vi "dfd_FXP PtByPt Cascaded SOS Form II.vi"(0 "x":T1={"value"=0, "wl"=0, "iwl"=0, "Signed"=TRUE} {"value" format="%.0x"}, 1 "coef b":i64[](array[numeric]), 2 "coef a":i64[](array[numeric]), 3 "#sec":i32, 5 "filtering statistics in":T4(array[cluster]) {"statistics information"."min value" format="%.2f"; "statistics information"."max value" format="%.2f"; "Quantizer Source" items=["Coefficients a/k"=0, "Coefficients b/v"=7, "Input"=1, "Output"=2, "Multiplicand"=3, "Product"=4, "Sum"=5, "Delay"=6]}, 6 "quantizers":T5[](array[typedef]) {"source" items=["Coef a/k"=0, "Coef b/v"=7, "Input"=1, "Output"=2, "Multiplicand"=3, "Product"=4, "Sum"=5, "Delay"=6, "Gain"=8]}, 7 "state in":i64[](array[numeric])) -> (13 "state out":i64[](array[numeric]), 14 "filtered x":T1={"value"=0, "wl"=0, "iwl"=0, "Signed"=TRUE} {"value" format="%.0x"}, 19 "filtering statistics out":T4(array[cluster]) {"statistics information"."min value" format="%.2f"; "statistics information"."max value" format="%.2f"; "Quantizer Source" items=["Coefficients a/k"=0, "Coefficients b/v"=7, "Input"=1, "Output"=2, "Multiplicand"=3, "Product"=4, "Sum"=5, "Delay"=6]})   [LabVIEW 2017, in "NI_DigFilter_FXP.lvlib"]
uses:
  <vilib>/addons/Digital Filter Design/NI_DigFilter_FXP.lvlib
  <vilib>/addons/Digital Filter Design/_Objects.llb/dfd_DFXP Data Type (scaler).ctl
  <vilib>/addons/Digital Filter Design/_Objects.llb/dfd_DFXP Operation Parameter.ctl
  <vilib>/addons/Digital Filter Design/_Objects.llb/dfd_Internal Quantization Srcs.ctl
  <vilib>/addons/Digital Filter Design/_Objects.llb/DFD Quantization Sources.ctl
  <vilib>/addons/Digital Filter Design/_Objects.llb/DFD FXP Statistics Data.ctl
  <vilib>/addons/Digital Filter Design/NI_DigFilterLicensed.lvlib
panel:
  in  "coef_a":T1={"value"=0, "wl"=0, "iwl"=0, "Signed"=TRUE} {"value" format="%.0x"}
  in  "coef_b":T1={"value"=0, "wl"=0, "iwl"=0, "Signed"=TRUE} {"value" format="%.0x"}
  in  "state":T1={"value"=0, "wl"=0, "iwl"=0, "Signed"=TRUE} {"value" format="%.0x"}
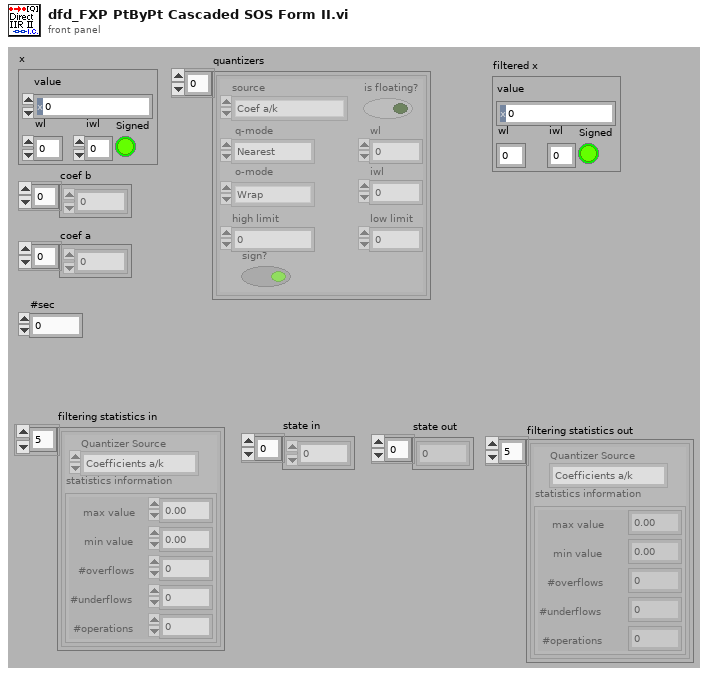
[diagram p1: front panel]
types:
  T1 = typedef "dfd_DFXP Data Type (scaler).ctl" = cluster{"value":i64, "wl":i16, "iwl":i16, "Signed":bool}
  T2 = typedef "NI_DigFilterLicensed.lvlib/DFD Quantization Sources.ctl" = u16
  T3 = typedef "NI_DigFilterLicensed.lvlib/DFD FXP Statistics Data.ctl" = cluster{"max value":ext, "min value":ext, "#overflows":i32, "#underflows":i32, "#operations":i32}
  T4 = cluster{"Quantizer Source":T2, "statistics information":T3}[]
  T5 = typedef "dfd_DFXP Operation Parameter.ctl" = cluster{"source":T6, "is floating?":bool, "o-mode":enum16{"Saturation", "Wrap"}, "q-mode":enum16{"Nearest", "Truncation"}, "wl":i16, "high limit":i64, "low limit":i64, "iwl":i16, "sign?":bool}
  T6 = typedef "NI_DigFilterLicensed.lvlib/dfd_Internal Quantization Srcs.ctl" = u16
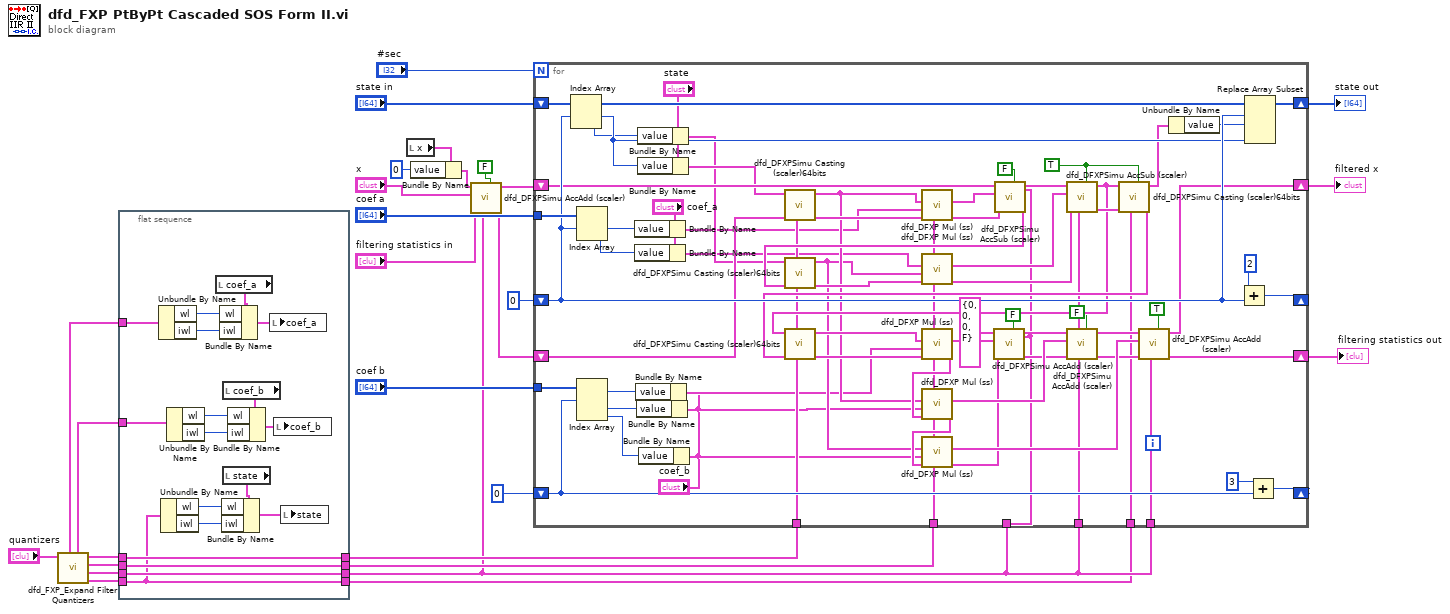
[diagram p0: block diagram]
diagram:
  n1 = call <vilib>:"dfd_FXP_Expand Filter Quantizers.vi"("FXPOPs"="quantizers") -> ("Delay"=w10:T5, "Sum"=w11:T5, "Product"=w12:T5, "Multiplicand"=w13:T5, "Coefficient b/v"=w9:T5, "Coefficient a/k"=w8:T5)  [unwired: 5 out]
  n2 = flat-sequence {
    tunnel: w10 -> [w29]
    tunnel: w13 -> [w42]
    tunnel: [w42] -> w7
    tunnel: [w41] -> w6
    tunnel: w12 -> [w41]
    tunnel: w11 -> [w40]
    tunnel: [w40] -> w5
    tunnel: [w29] -> _
    tunnel: w9 -> [w38]
    tunnel: w8 -> [w32]
    tunnel: [w29] -> w4
    frame #0 {
      n3 = Unbundle By Name(w32) -> ("wl"=w34:i16, "iwl"=w33:i16)
      n4 = Unbundle By Name(w29) -> ("wl"=w45:i16, "iwl"=w44:i16)
      n5 = Unbundle By Name(w38) -> ("wl"=w35:i16, "iwl"=w39:i16)
      n6 = local read "coef_a"() -> (w30:T1)
      n7 = Bundle By Name(cluster=w30, "wl"=w34, "iwl"=w33) -> (w31:T1)
      n8 = local read "coef_b"() -> (w36:T1)
      n9 = local read "state"() -> (w46:T1)
      n10 = Bundle By Name(cluster=w46, "wl"=w45, "iwl"=w44) -> (w43:T1)
      n11 = Bundle By Name(cluster=w36, "wl"=w35, "iwl"=w39) -> (w37:T1)
      n12 = local write "coef_a"(w31) -> ()
      n13 = local write "coef_b"(w37) -> ()
      n14 = local write "state"(w43) -> ()
    }
  }
  n15 = local read "x"() -> (w3:T1)
  n16 = Bundle By Name(cluster=w3, "value"=i64 0) -> (w1:T1)
  n17 = call <vilib>:"dfd_DFXPSimu AccAdd (scaler).vi"("quantize output? (T)"=FALSE ("quantize output?"), "op params"=w5, "filtering statistics in"="filtering statistics in", "addend"="x", "acc in"=w1) -> ("filtering statistics out"=w16:T4, "acc out"=w18:T1)  [unwired: 5 out]
  n18 = for {
    N: "#sec" -> [_]
    shift-right: [w115] -> w27
    shift-left: "state in" -> [w116]
    shift-right: [w114] -> _
    shift-left: 0 -> [w108]
    shift-right: [w103] -> w21
    shift-left: w18 -> [w106]
    shift-right: [w111] -> _
    shift-left: 0 -> [w107]
    tunnel: "coef a" -> [w110]
    tunnel: "coef b" -> [w109]
    tunnel: w7 -> [w81]
    tunnel: w6 -> [w80]
    tunnel: w5 -> [w76]
    tunnel: w4 -> [w74]
    tunnel: w5 -> [w75]
    shift-right: [w83] -> w19
    shift-left: w16 -> [w95]
    tunnel: w5 -> [w73]
    w58 = TRUE ("quantize output?")
    n19 = Index Array(array=w116, index #1=w108) -> (element #1=w98:i64, element #2=w97:i64)  [unwired: 1 in]
    n20 = Index Array(array=w110, index #1=w108) -> (element #1=w70:i64, element #2=w69:i64)  [unwired: 1 in]
    n21 = Index Array(array=w109, index #1=w107) -> (element #1=w67:i64, element #2=w65:i64, element #3=w63:i64)  [unwired: 2 in]
    n22 = Bundle By Name(cluster="coef_a", "value"=w70) -> (w53:T1)
    n23 = Bundle By Name(cluster="coef_a", "value"=w69) -> (w52:T1)
    n24 = Bundle By Name(cluster="coef_b", "value"=w67) -> (w50:T1)
    n25 = Bundle By Name(cluster="coef_b", "value"=w65) -> (w49:T1)
    n26 = Bundle By Name(cluster="state", "value"=w97) -> (w56:T1)
    n27 = Bundle By Name(cluster="state", "value"=w98) -> (w57:T1)
    n28 = Bundle By Name(cluster="coef_b", "value"=w63) -> (w48:T1)
    n29 = call <vilib>:"dfd_DFXPSimu Casting (scaler)64bits.vi"("op params"=w81, "filtering statistics in"=w95, "Value in"=w57) -> ("filtering statistics out"=w94:T4, "Value out"=w66:T1)  [unwired: 1 in, 6 out]
    n30 = call <vilib>:"dfd_DFXP Mul (ss).vi"("op params"=w80, "filtering statistics in"=w94, "Value in 2"=w53, "Value in"=w66) -> ("filtering statistics out"=w92:T4, "Value out"=w102:T1)  [unwired: 6 out]
    n31 = call <vilib>:"dfd_DFXPSimu AccSub (scaler).vi"("quantize output?(T)"=FALSE, "op params"=w76, "filtering statistics in"=w92, "addend"=w102, "acc in"=w106) -> ("filtering statistics out"=w91:T4, "acc out"=w105:T1)  [unwired: 5 out]
    n32 = call <vilib>:"dfd_DFXPSimu Casting (scaler)64bits.vi"("op params"=w81, "filtering statistics in"=w91, "Value in"=w56) -> ("filtering statistics out"=w93:T4, "Value out"=w64:T1)  [unwired: 1 in, 6 out]
    n33 = call <vilib>:"dfd_DFXP Mul (ss).vi"("op params"=w80, "filtering statistics in"=w93, "Value in 2"=w64, "Value in"=w52) -> ("filtering statistics out"=w87:T4, "Value out"=w101:T1)  [unwired: 6 out]
    n34 = call <vilib>:"dfd_DFXPSimu AccSub (scaler).vi"("quantize output?(T)"=w58, "op params"=w75, "filtering statistics in"=w87, "addend"=w101, "acc in"=w105) -> ("filtering statistics out"=w86:T4, "acc out"=w82:T1)  [unwired: 5 out]
    n35 = call <vilib>:"dfd_DFXPSimu Casting (scaler)64bits.vi"("quantize output?(T)"=w58, "op params"=w74, "filtering statistics in"=w86, "Value in"=w82) -> ("filtering statistics out"=w85:T4, "Value out"=w96:T1)  [unwired: 6 out]
    n36 = call <vilib>:"dfd_DFXPSimu Casting (scaler)64bits.vi"("op params"=w81, "filtering statistics in"=w85, "Value in"=w82) -> ("filtering statistics out"=w90:T4, "Value out"=w68:T1)  [unwired: 1 in, 6 out]
    n37 = call <vilib>:"dfd_DFXP Mul (ss).vi"("op params"=w80, "filtering statistics in"=w90, "Value in 2"=w50, "Value in"=w68) -> ("filtering statistics out"=w89:T4, "Value out"=w72:T1)  [unwired: 6 out]
    n38 = call <vilib>:"dfd_DFXP Mul (ss).vi"("op params"=w80, "filtering statistics in"=w89, "Value in 2"=w49, "Value in"=w66) -> ("filtering statistics out"=w88:T4, "Value out"=w100:T1)  [unwired: 6 out]
    n39 = call <vilib>:"dfd_DFXP Mul (ss).vi"("op params"=w80, "filtering statistics in"=w88, "Value in 2"=w48, "Value in"=w64) -> ("filtering statistics out"=w78:T4, "Value out"=w99:T1)  [unwired: 6 out]
    n40 = call <vilib>:"dfd_DFXPSimu AccAdd (scaler).vi"("quantize output? (T)"=FALSE ("quantize output?"), "op params"=w76, "filtering statistics in"=w78, "addend"=w72, "acc in"=T1 {"value"=0, "wl"=0, "iwl"=0, "Signed"=FALSE}) -> ("filtering statistics out"=w77:T4, "acc out"=w79:T1)  [unwired: 5 out]
    n41 = call <vilib>:"dfd_DFXPSimu AccAdd (scaler).vi"("quantize output? (T)"=FALSE ("quantize output?"), "op params"=w75, "filtering statistics in"=w77, "addend"=w100, "acc in"=w79) -> ("filtering statistics out"=w84:T4, "acc out"=w104:T1)  [unwired: 5 out]
    n42 = call <vilib>:"dfd_DFXPSimu AccAdd (scaler).vi"("quantize output? (T)"=TRUE ("quantize output?"), "op params"=w73, "filtering statistics in"=w84, "addend"=w99, "acc in"=w104) -> ("filtering statistics out"=w83:T4, "acc out"=w103:T1)  [unwired: 5 out]
    n43 = Unbundle By Name(w96) -> ("value"=w54:i64)
    n44 = Add(x=2 ("y"), y=w108) -> (x+y=w114:i32)
    n45 = Replace Array Subset(array=w116, new element #1=w54, index #1=w108, new element #2=w98) -> (w115:i64[])  [unwired: 1 in]
    n46 = Add(x=3, y=w107) -> (x+y=w111:i32)
  }
  "filtered x" <- w21
  "state out" <- w27
  "filtering statistics out" <- w19
